vi "camera globals - SubVI.vi"() -> ()   [LabVIEW 2014]
uses:
  Glimpse-master/Microscope plugins/ixon camera/andor camera properties.ctl
panel:
  in  "Camera Properties":T1
  in  "Number of acquisition blocks":i8(slide)=10 scale=0.0..20.0
  in  "Camera Acquiring":bool
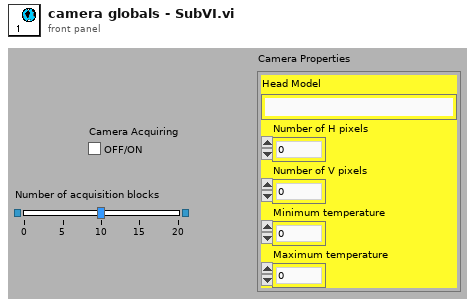
[diagram p1: front panel]
types:
  T1 = typedef "andor camera properties.ctl" = cluster{"Head Model":string, "Number of H pixels":i32, "Number of V pixels":i32, "Minimum temperature":i32, "Maximum temperature":i32}
diagram:
